vi "Uninit.vi"(11 "Event Msg Type Strategy in":refnum<class "Event Msg Type Strategy.lvclass">) -> (0 "error out":errorcluster)   [LabVIEW 2021, in "jettl.lvlib" / "Msg Type Strategy.lvlib" / "Event Msg Type Strategy.lvclass"]
uses:
  Event Msg Type Strategy.lvclass
  Event Msg Type Strategy.lvclass/Event Msg Type Strategy.ctl
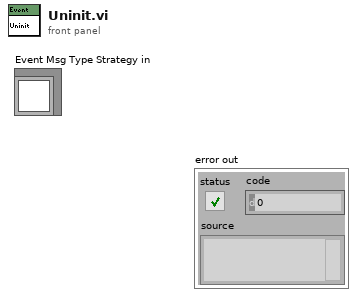
[diagram p1: front panel]
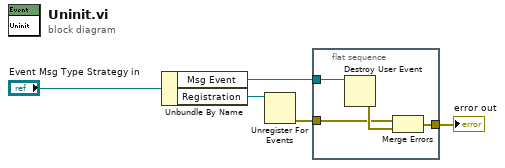
[diagram p0: block diagram]
diagram:
  n1 = Unbundle By Name("Event Msg Type Strategy in") -> ("Msg Event"=w4:refnum<user-event>, "Registration"=w3:refnum<event-registration>)
  n2 = Unregister For Events(event registration refnum=w3) -> (error out=w1:errorcluster)  [unwired: 1 in]
  n3 = flat-sequence {
    tunnel: w4 -> [w9]
    tunnel: [w8] -> w2
    tunnel: w1 -> [w6]
    frame #0 {
      n4 = Destroy User Event(user event=w9) -> (error out=w7:errorcluster)  [unwired: 1 in]
      n5 = Merge Errors(w6, w7) -> (w8:errorcluster)
    }
  }
  "error out" <- w2
